vi "Set_Data.vi"(8 "error in (no error)":errorcluster caption="entrée d'erreur (pas d'erreur)", 11 "Firebase Benches en entrée":refnum<class "Firebase Benches P2193.lvclass">) -> (0 "error out":errorcluster caption="sortie d'erreur", 3 "Firebase Benches en sortie":refnum<class "Firebase Benches P2193.lvclass">)   [LabVIEW 2020, in "Library Instrument & Equipement.lvlib" / "Library FireBase.lvlib" / "Firebase Benches P2193.lvclass"]
doc: "Create New document\nPlease initialise the following values\n - Name BDD\n - Document\n - API Key"
uses:
  Firebase Benches P2193.lvclass
  C:/Users/ngarcin/OneDrive - Altyor/Standard TB/Class/Firebase/Source/Firebase Altyor/Firebase Altyor.lvclass
  C:/Users/ngarcin/OneDrive - Altyor/Standard TB/Class/Firebase/Source/Firebase Driver/Firebase Driver.lvclass
  Firebase Benches P2193.lvclass/Firebase Benches P2193.ctl
  Firebase Altyor/Firebase Altyor.lvclass
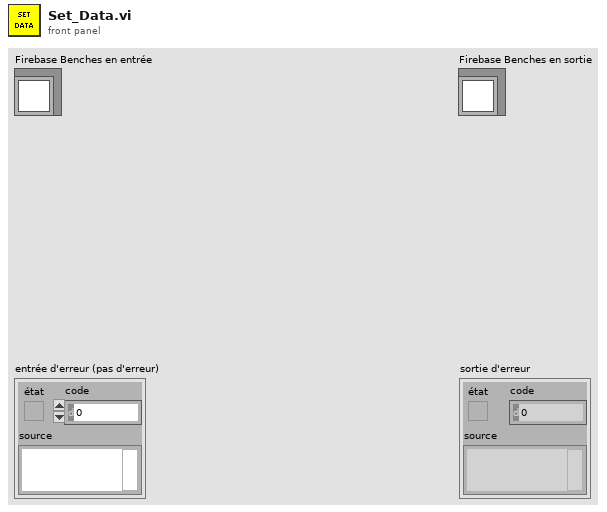
[diagram p1: front panel]
types:
  T1 = cluster{"Result":cluster{"booleanValue":bool}, "CreationDate":cluster{"timestampValue":string}, "Batch":cluster{"stringValue":string}, "SerialNumber":cluster{"stringValue":string}, "EndOfProduction":cluster{"timestampValue":string}, "FW_Version":cluster{"mapValue":cluster{"fields":cluster{"Bootloader":cluster{"mapValue":cluster{"fields":cluster{"File_Name":cluster{"stringValue":string}, "Version":cluster{"mapValue":cluster{"fields":cluster{"Major":cluster{"stringValue":string}, "Minor":cluster{"stringValue":string}}}}, "Checksum":cluster{"stringValue":string}}}}, "SoftDevice":cluster{"mapValue":cluster{"fields":cluster{"File_Name":cluster{"stringValue":string}, "Version":cluster{"mapValue":cluster{"fields":cluster{"Major":cluster{"stringValue":string}, "Minor":cluster{"stringValue":string}}}}, "Checksum":cluster{"stringValue":string}}}}, "DFU":cluster{"mapValue":cluster{"fields":cluster{"File_Name":cluster{"stringValue":string}, "Version":cluster{"mapValue":cluster{"fields":cluster{"Major":cluster{"stringValue":string}, "Minor":cluster{"stringValue":string}}}}, "Checksum":cluster{"stringValue":string}}}}}}}, "PartNumber":cluster{"stringValue":string}, "OrderNumber":cluster{"stringValue":string}, "Operator":cluster{"stringValue":string}, "SN_CPU":cluster{"stringValue":string}}
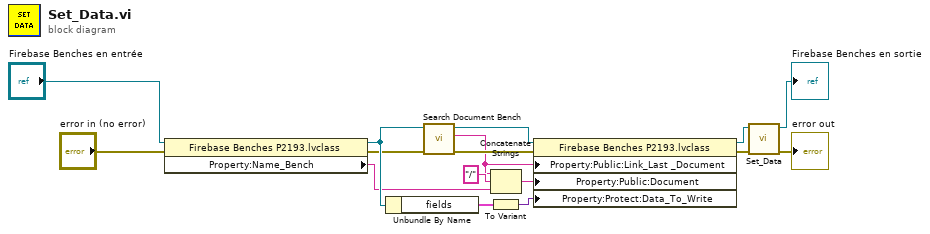
[diagram p0: block diagram]
diagram:
  n1 = property class="Firebase Benches P2193.lvclass"(reference="Firebase Benches en entrée", error in="error in (no error)") -> (reference out=w4:refnum<class "Firebase Benches P2193.lvclass">, error out=w2:errorcluster, "Property:Name_Bench"=w1:string)
  n2 = Unbundle By Name(w4) -> ("fields"=w12:T1)
  n3 = call "Search Document Bench.vi"("entrée d'erreur (pas d'erreur)"=w2, "Firebase Altyor en entrée"=w4) -> ("sortie d'erreur"=w10:errorcluster, "Source"=w6:string, "Firebase Altyor en sortie"=w9:refnum<class "Firebase Benches P2193.lvclass">)  [unwired: 7 in]
  n4 = Concatenate Strings(w6, "/" ("chaîne"), w1) -> (w7:string)
  n5 = To Variant(anything=w12) -> (Variant=w8:variant)
  n6 = property class="Firebase Benches P2193.lvclass"(reference=w9, error in=w10, "Property:Public:Link_Last _Document"=w6, "Property:Public:Document"=w7, "Property:Protect:Data_To_Write"=w8) -> (reference out=w14:refnum<class "Firebase Benches P2193.lvclass">, error out=w13:errorcluster)
  n7 = call-parent "Set_Data.vi"("error in (no error)"=w13, "Firebase Altyor en entrée"=w14) -> ("error out"=→"error out":errorcluster, "Firebase Altyor en sortie"=→"Firebase Benches en sortie":refnum<class "Firebase Benches P2193.lvclass">)  [unwired: 8 in]
